vi "Coerce Steering Frame Velocity.vi"(8 "error in (no error)":errorcluster, 10 "steering frame velocity":dbl[](array[numeric])=[0.0, 0.0, 0.0], 11 "steering frame in":refnum<class "NI_Robotics_Steering Frame.lvclass">) -> (0 "error out":errorcluster, 2 "coerced steering frame velocity":dbl[](array[numeric]), 3 "steering frame out":refnum<class "NI_Robotics_Steering Frame.lvclass">)   [LabVIEW 2017, in "NI_Robotics_Steering Frame.lvclass"]
doc: "Coerces the steering frame velocity to meet the constraints of the steering frame type. This VI does not coerce the velocity based on the constraints of individual wheels."
uses:
  <vilib>/robotics/Steering/Steering Frame/NI_Robotics_Steering Frame.lvclass
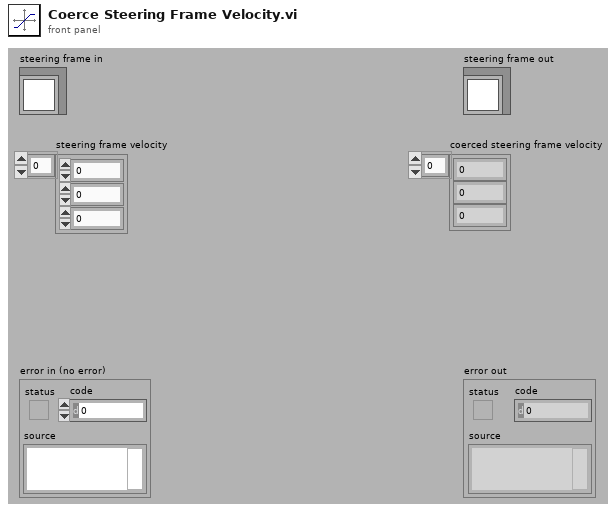
[diagram p1: front panel]
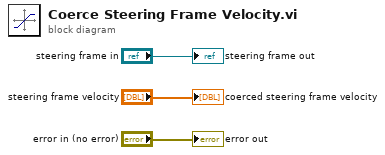
[diagram p0: block diagram]
diagram:
  "error out" <- "error in (no error)"
  "steering frame out" <- "steering frame in"
  "coerced steering frame velocity" <- "steering frame velocity"
